vi "saveTuner.vi"(0 "configuration file path":path=path "C:/users/develoer/desktop/foo.ini", 5 "hue":cluster{dbl, dbl}(slide)={0.0, 4.747474747474747} scale=0.0..10.0, 7 "sat":cluster{dbl, dbl}(slide)={0.0, 4.747474747474747} scale=0.0..10.0, 9 "val":cluster{dbl, dbl}(slide)={0.0, 4.747474747474747} scale=0.0..10.0, 11 "error in (no error)":errorcluster) -> (15 "error out":errorcluster)   [LabVIEW 2016]
uses:
  <vilib>/Utility/config.llb/Write Key (Double).vi
  <vilib>/Utility/config.llb/NI_LVConfig.lvlib
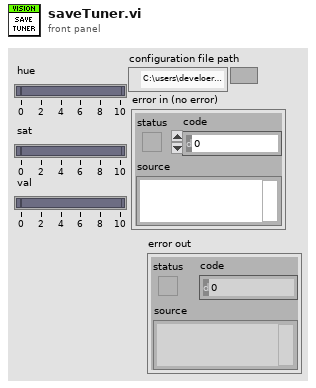
[diagram p1: front panel]
types:
  T1 = typedef "NI_LVConfig.lvlib/Config Data RefNum.ctl" = refnum<k1>
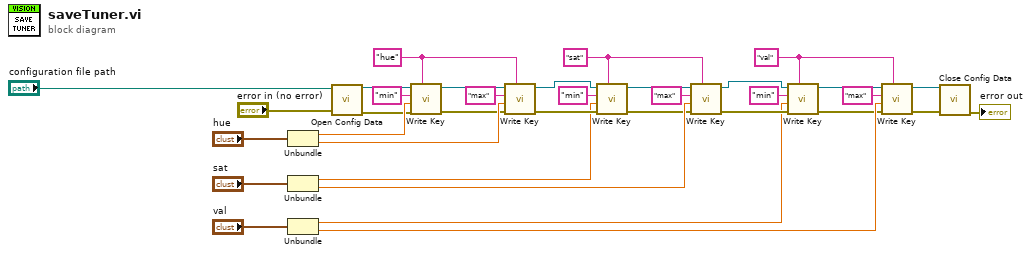
[diagram p0: block diagram]
diagram:
  w18 = "val" ("section")
  w22 = "sat" ("section")
  w23 = "hue" ("section")
  n1 = Unbundle("hue") -> (w32:dbl, w29:dbl)
  n2 = Unbundle("sat") -> (w20:dbl, w19:dbl)
  n3 = Unbundle("val") -> (w11:dbl, w10:dbl)
  n4 = call <vilib>:"Open Config Data.vi"("error in (no error)"="error in (no error)", "configuration file path"="configuration file path") -> ("error out"=w6:errorcluster, "refnum"=w35:T1)  [unwired: 7 in, 1 out]
  n5 = call-poly <vilib>:"Write Key.vi"("section"=w23, "error in (no error)"=w6, "value"=w32, "key"="min", "refnum"=w35) -> ("error out"=w5:errorcluster, "refnum out"=w30:T1)  [unwired: 4 in, 1 out]
  n6 = call-poly <vilib>:"Write Key.vi"("section"=w23, "error in (no error)"=w5, "value"=w29, "key"="max", "refnum"=w30) -> ("error out"=w24:errorcluster, "refnum out"=w25:T1)  [unwired: 4 in, 1 out]
  n7 = call-poly <vilib>:"Write Key.vi"("section"=w22, "error in (no error)"=w24, "value"=w20, "key"="min", "refnum"=w25) -> ("error out"=w8:errorcluster, "refnum out"=w28:T1)  [unwired: 4 in, 1 out]
  n8 = call-poly <vilib>:"Write Key.vi"("section"=w22, "error in (no error)"=w8, "value"=w19, "key"="max", "refnum"=w28) -> ("error out"=w14:errorcluster, "refnum out"=w13:T1)  [unwired: 4 in, 1 out]
  n9 = call-poly <vilib>:"Write Key.vi"("section"=w18, "error in (no error)"=w14, "value"=w11, "key"="min", "refnum"=w13) -> ("error out"=w7:errorcluster, "refnum out"=w15:T1)  [unwired: 4 in, 1 out]
  n10 = call-poly <vilib>:"Write Key.vi"("section"=w18, "error in (no error)"=w7, "value"=w10, "key"="max", "refnum"=w15) -> ("error out"=w4:errorcluster, "refnum out"=w3:T1)  [unwired: 4 in, 1 out]
  n11 = call <vilib>:"Close Config Data.vi"("error in (no error)"=w4, "refnum"=w3) -> ("error out"=→"error out":errorcluster)  [unwired: 8 in, 1 out]
